vi "Knock Sensor Constructor.vi"(8 "error in (no error)":errorcluster, 10 "Generate Signal Path":path, 11 "Signal Parameters":string) -> (0 "error out":errorcluster, 3 "EST Knock Sensor.lvclass":refnum<class "Knock Sensor.lvclass">)   [LabVIEW 2015, in "Knock Sensor.lvclass"]
uses:
  Knock Sensor.lvclass
  Knock Sensor.lvclass/Knock Sensor.ctl
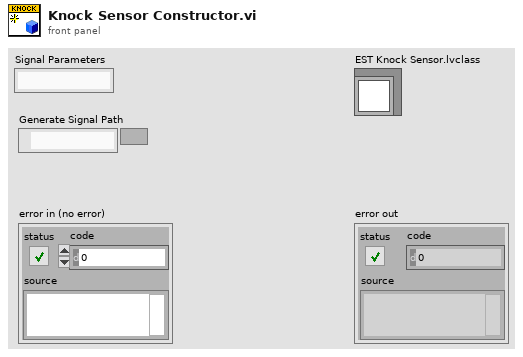
[diagram p1: front panel]
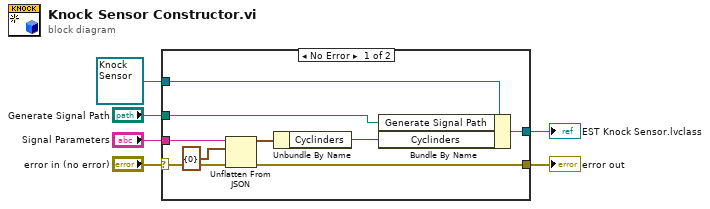
[diagram p0: block diagram]
diagram:
  n1 = case shown="No Error" "error in (no error)" {
    selector: "error in (no error)" -> [w11 w17]
    tunnel: "Generate Signal Path" -> [w10 _]
    tunnel: "Signal Parameters" -> [w15 _]
    tunnel: [w9 w17] -> w3
    tunnel: [w8 w16] -> w2
    tunnel: refnum<class "Knock Sensor.lvclass"> refnum ("EST Knock Sensor.lvclass") -> [w7 w16]
    frame No Error {
      n2 = Unflatten From JSON(JSON string=w15, type and defaults=cluster{"Cyclinders":u32} {"Cyclinders"=0}, error in (no error)=w11) -> (value=w13:cluster{"Cyclinders":u32}, error out=w9:errorcluster)  [unwired: 4 in]
      n3 = Unbundle By Name(w13) -> ("Cyclinders"=w12:u32)
      n4 = Bundle By Name(cluster=w7, "Generate Signal Path"=w10, "Cyclinders"=w12) -> (w8:refnum<class "Knock Sensor.lvclass">)
    }
    frame Error {
    }
  }
  "error out" <- w3
  "EST Knock Sensor.lvclass" <- w2
